vi "Start.vi"(8 "error in (no error)":errorcluster, 9 "Duration (s)":dbl, 10 "Set Fire (%)":dbl min=0.0 max=100.0 format="%.2f %", 11 "Direct Cooker in":refnum<class "Direct Cooker.lvclass">) -> (0 "error out":errorcluster, 3 "Direct Cooker out":refnum<class "Direct Cooker.lvclass">)   [LabVIEW 2024, in "Cooker Actor.lvlib" / "Direct Cooker.lvclass"]
uses:
  Direct Cooker.lvclass
  Direct Cooker.lvclass/Direct Cooker.ctl
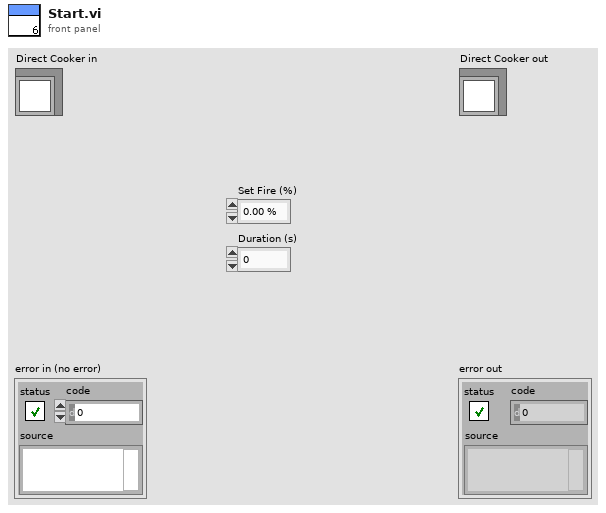
[diagram p1: front panel]
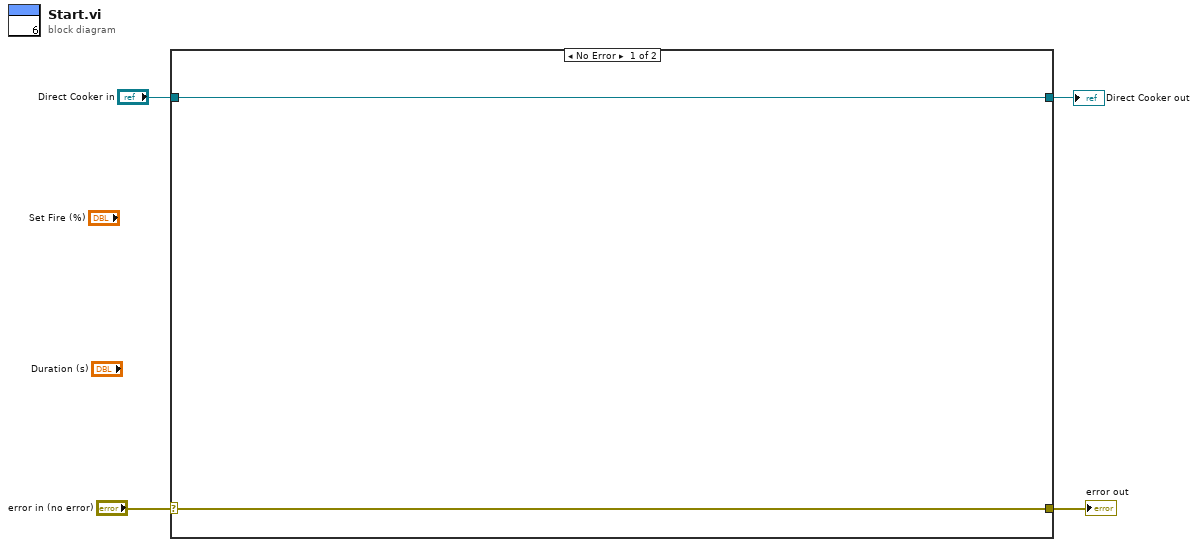
[diagram p0: block diagram]
diagram:
  n1 = case shown="No Error" "error in (no error)" {
    selector: "error in (no error)" -> [w6 w7]
    tunnel: [w6 w7] -> w3
    tunnel: "Direct Cooker in" -> [w5 w8]
    tunnel: [w5 w8] -> w1
    frame No Error {
    }
    frame Error {
    }
  }
  "error out" <- w3
  "Direct Cooker out" <- w1
